vi "PH_Stepmotor_BaseClass.Waveplate - Percent 2 Angle.vi"(1 "rel. Intensity [%]":dbl) -> (0 "Angle [°]":dbl format="%#.1g")   [LabVIEW 2014, in "PH_Stepmotor_BaseClass.lvlib"]
doc: "This VI calculalates the waveplate Angle (in degrees) for a given relative Intensity (in percent, coerced to the range between 0 and 100%) by\n\nAngle [°] = arcsin (sqrt (rel. Intensity [%] / 100) ) / 2\n\nThe result is rounded to 1 digit after the decimal point."
uses:
  PH_Stepmotor_BaseClass.lvlib
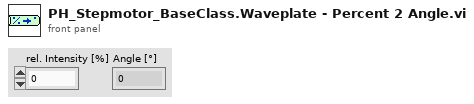
[diagram p1: front panel]
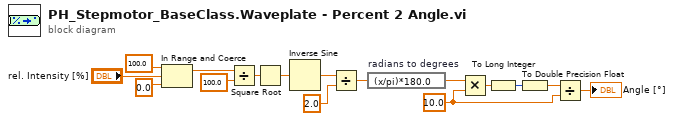
[diagram p0: block diagram]
diagram:
  w1 = 10.0 ("y")
  n1 = In Range and Coerce(upper limit=100.0, x="rel. Intensity [%]", lower limit=0.0) -> (coerced(x)=w8:dbl)  [unwired: 1 out]
  n2 = Divide(x=w8, y=100.0) -> (x/y=w15:dbl)
  n3 = Square Root(x=w15) -> (sqrt(x)=w10:dbl)
  n4 = Inverse Sine(1:w10) -> (0:w12:dbl)
  n5 = Divide(x=w12, y=2.0) -> (x/y=w11:dbl)
  n6 = expression code="(x/pi)*180.0" "radians to degrees"(w11) -> (w9:dbl)
  n7 = Multiply(x=w9, y=w1) -> (x*y=w5:dbl)
  n8 = To Long Integer(number=w5) -> (32bit integer=w4:i32)
  n9 = To Double Precision Float(number=w4) -> (double precision float=w3:dbl)
  n10 = Divide(x=w3, y=w1) -> (x/y=→"Angle [°]":dbl)
